vi "sr510_poll.vi"(5 "error in":errorcluster) -> (0 "error out":errorcluster, 1 "Time constant [s]":string, 2 "Phase":string, 3 "Sensitivity [mV]":string, 4 "Locked":bool)   [LabVIEW 2012]
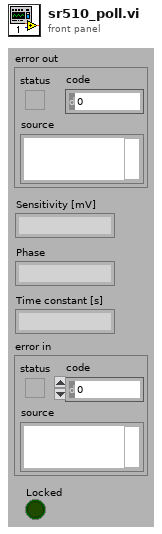
[diagram p1: front panel]
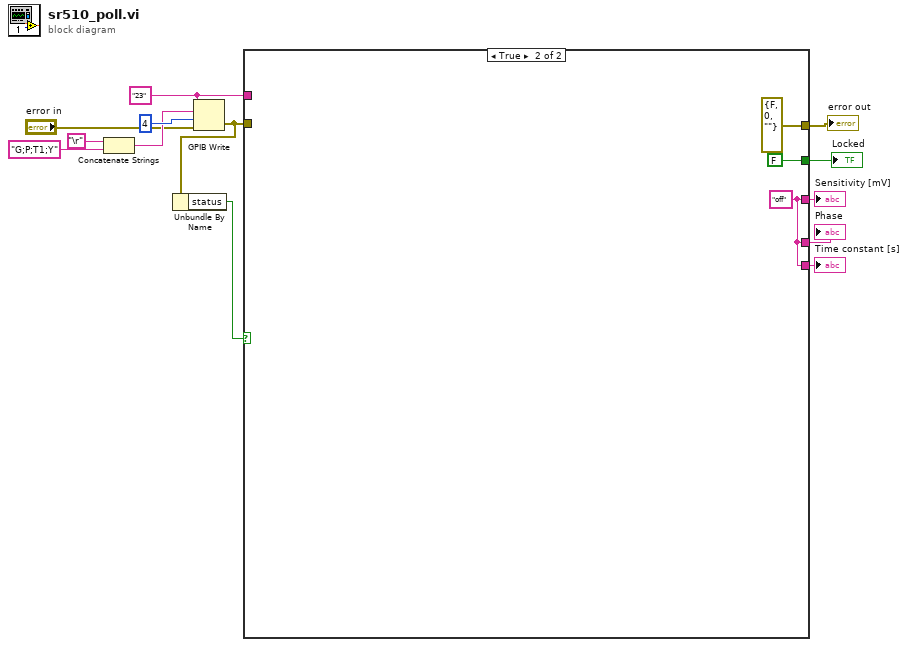
[diagram p0: block diagram]
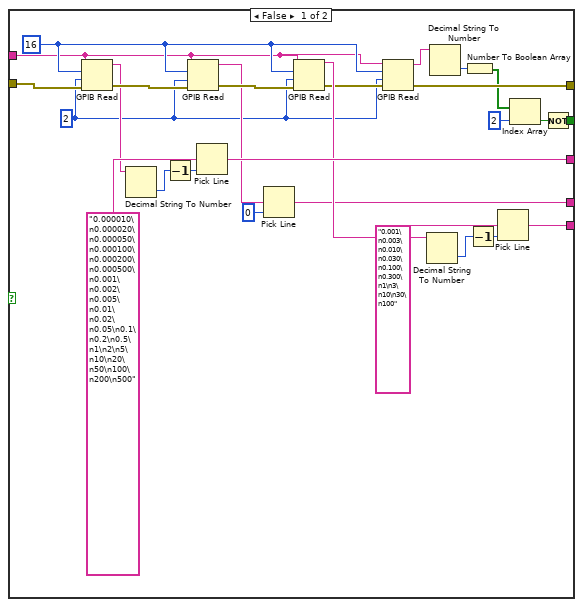
[diagram p2: hidden frame]
diagram:
  w3 = "23" ("address string")
  n1 = Concatenate Strings("\r", "G;P;T1;Y" ("data")) -> (w12:string)
  n2 = GPIB Write(0:w3, 1:w12, 2:i16 4 ("mode (0)"), 3:"error in") -> (6:w2:errorcluster)  [unwired: 1 in, 1 out]
  n3 = Unbundle By Name(w2) -> ("status"=w1:bool)
  n4 = case shown="True" w1 {
    tunnel: w2 -> [w40 _]
    tunnel: [w34 w41] -> w8
    tunnel: [w30 w41] -> w7
    tunnel: [w28 w41] -> w6
    tunnel: [w22 FALSE] -> w5
    tunnel: [w20 errorcluster {"status"=FALSE, "code"=0, "source"=""} ("error out")] -> w4
    tunnel: w3 -> [w18 _]
    frame False {
      w19 = 16 ("byte count")
      w17 = i16 2 ("mode (0)")
      n5 = GPIB Read(0:w18, 1:w19, 2:w17, 3:w40) -> (5:w36:string, 7:w39:errorcluster)  [unwired: 1 in, 1 out]
      n6 = Decimal String To Number(string=w36) -> (number=w35:i32)  [unwired: 2 in, 1 out]
      n7 = Decrement(x=w35) -> (x-1=w26:i32)
      n8 = GPIB Read(0:w18, 1:w19, 2:w17, 3:w39) -> (5:w29:string, 7:w38:errorcluster)  [unwired: 1 in, 1 out]
      n9 = Pick Line(multi-line string="0.000010\n0.000020\n0.000050\n0.000100\n0.000200\n0.000500\n0.001\n0.002\n0.005\n0.01\n0.02\n0.05\n0.1\n0.2\n0.5\n1\n2\n5\n10\n20\n50\n100\n200\n500", line index=w26) -> (output string=w34:string)  [unwired: 1 in]
      n10 = Pick Line(multi-line string=w29, line index=0) -> (output string=w28:string)  [unwired: 1 in]
      n11 = GPIB Read(0:w18, 1:w19, 2:w17, 3:w38) -> (5:w31:string, 7:w21:errorcluster)  [unwired: 1 in, 1 out]
      n12 = GPIB Read(0:w18, 1:w19, 2:w17, 3:w21) -> (5:w16:string, 7:w20:errorcluster)  [unwired: 1 in, 1 out]
      n13 = Decimal String To Number(string=w31) -> (number=w33:i32)  [unwired: 2 in, 1 out]
      n14 = Decimal String To Number(string=w16) -> (number=w15:i32)  [unwired: 2 in, 1 out]
      n15 = Number To Boolean Array(number=w15) -> (Boolean array=w14:bool[])
      n16 = Decrement(x=w33) -> (x-1=w25:i32)
      n17 = Pick Line(multi-line string="0.001\n0.003\n0.010\n0.030\n0.100\n0.300\n1\n3\n10\n30\n100", line index=w25) -> (output string=w30:string)  [unwired: 1 in]
      n18 = Index Array(array=w14, index=2) -> (element=w23:bool)
      n19 = Not(x=w23) -> (.not. x?=w22:bool)
    }
    frame True {
      w41 = "off" ("output string")
    }
  }
  "Sensitivity [mV]" <- w8
  "Phase" <- w6
  "Time constant [s]" <- w7
  "error out" <- w4
  "Locked" <- w5
